vi "2d queue - Copia.vi"() -> ()   [LabVIEW 2020]
uses:
  control/Data Form.ctl
  control/fgv.ctl
  control/file structure.ctl
  <vilib>/Analysis/1siggen.llb/Ramp Pattern by Samples.vi
  queue/Front Panel Message Queue.lvlib
  <vilib>/Analysis/NI_AALBase.lvlib
panel:
  out "XY Graph":cluster{"Ramp Pattern":dbl[], dbl[]}(graph)
  out "Data Loaded":dbl[][](array[numeric])
  out "Data Form":T1
  out "error out":errorcluster
  in  "error in":errorcluster
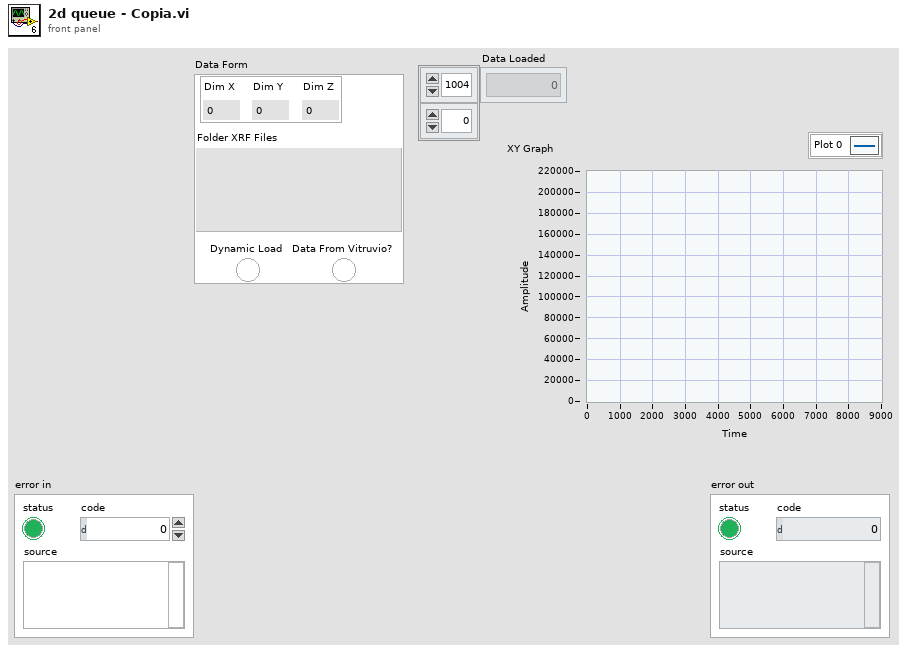
[diagram p1: front panel]
types:
  T1 = typedef "Data Form.ctl" = cluster{"Dimensions":cluster{"Dim X":i32, "Dim Y":i32, "Dim Z":i32}, "Folder XRF Files":path, "Dynamic Load":bool, "Data From Vitruvio?":bool}
  T2 = typedef "Front Panel Message Queue.lvlib/2d3d Message Queues.ctl" = cluster{"Main":refnum<queue>, "2d":refnum<queue>, "3d":refnum<queue>}
  T3 = typedef "fgv.ctl" = enum16{"initialize", "get data", "set data"}
  T4 = typedef "file structure.ctl" = cluster{"Colonna":i32, "Offset Righe":i32, "Coda Righe":i32, "Transpose":bool}
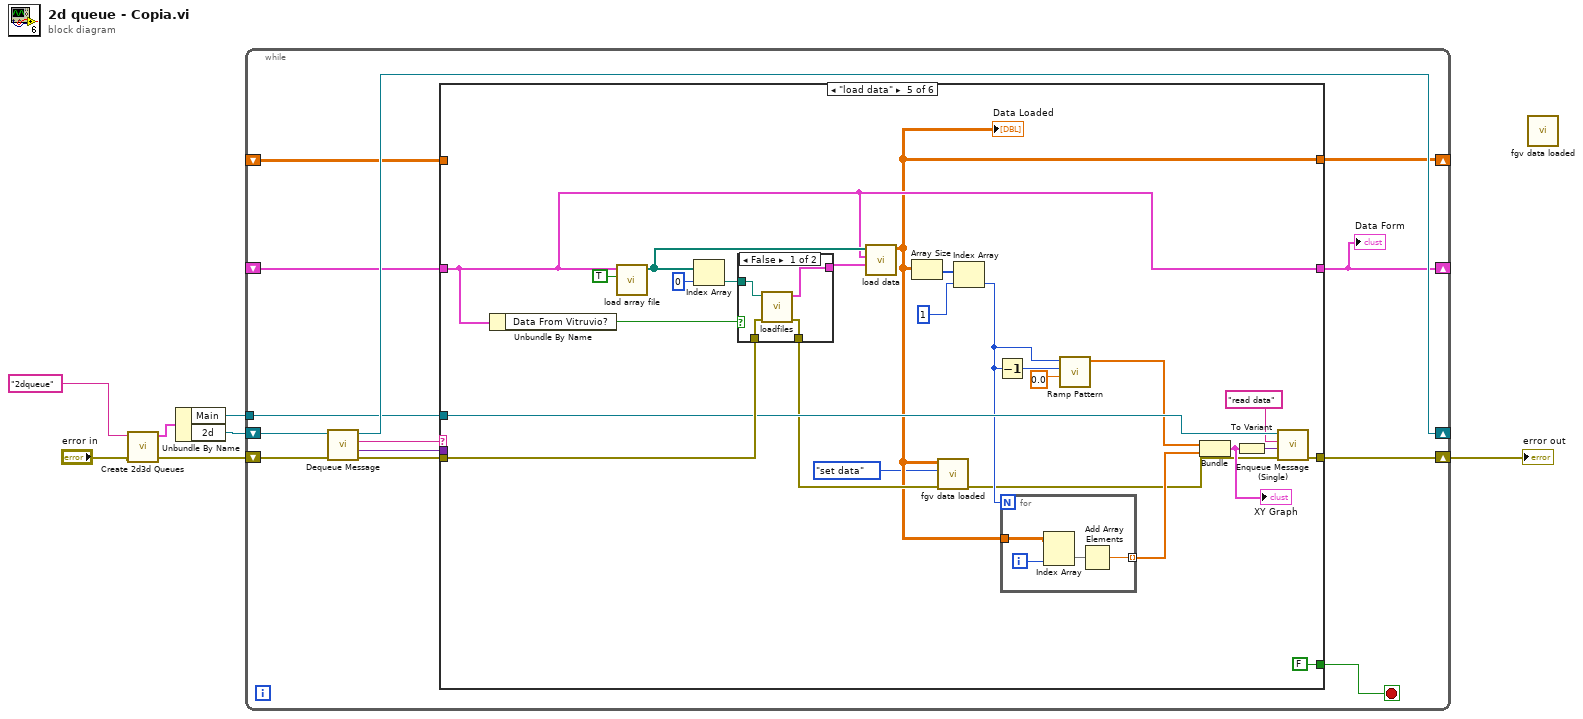
[diagram p0: block diagram]
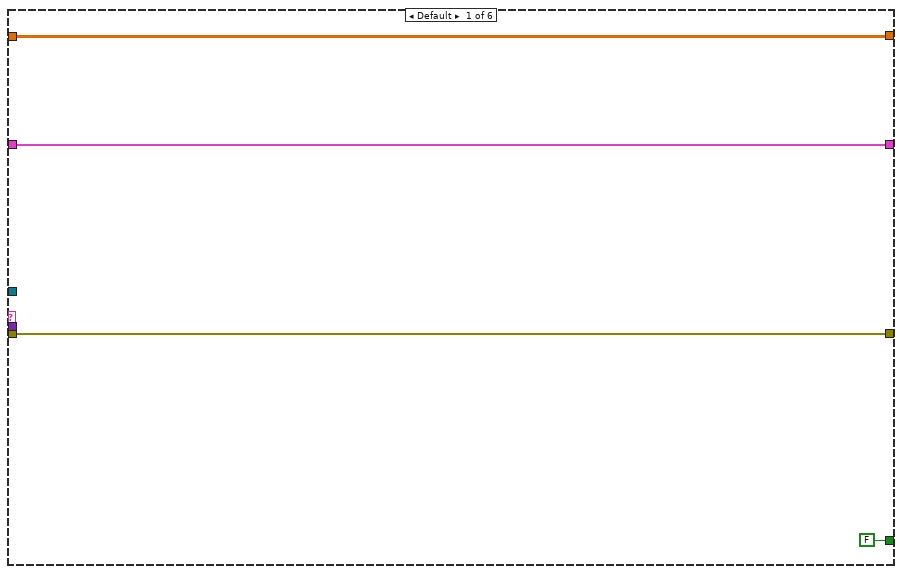
[diagram p2: hidden frame]
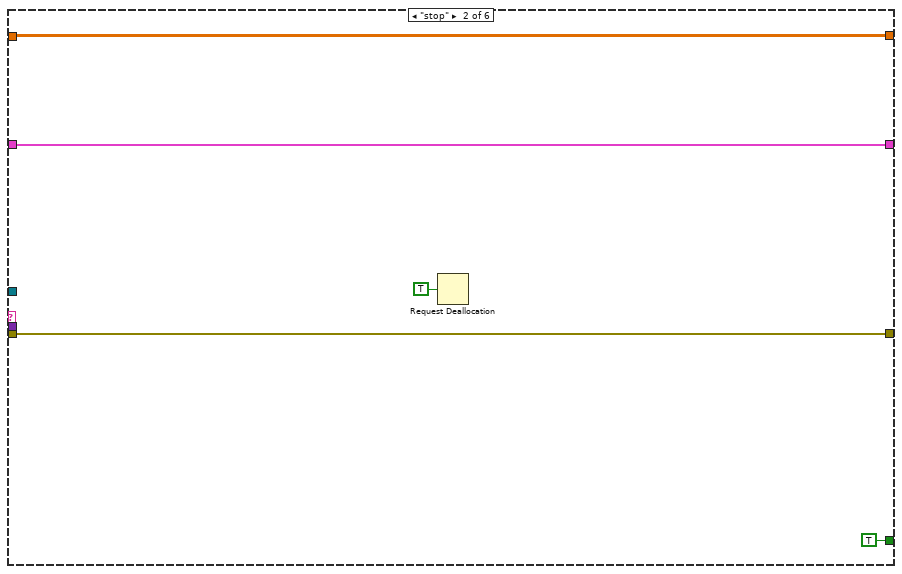
[diagram p3: hidden frame]
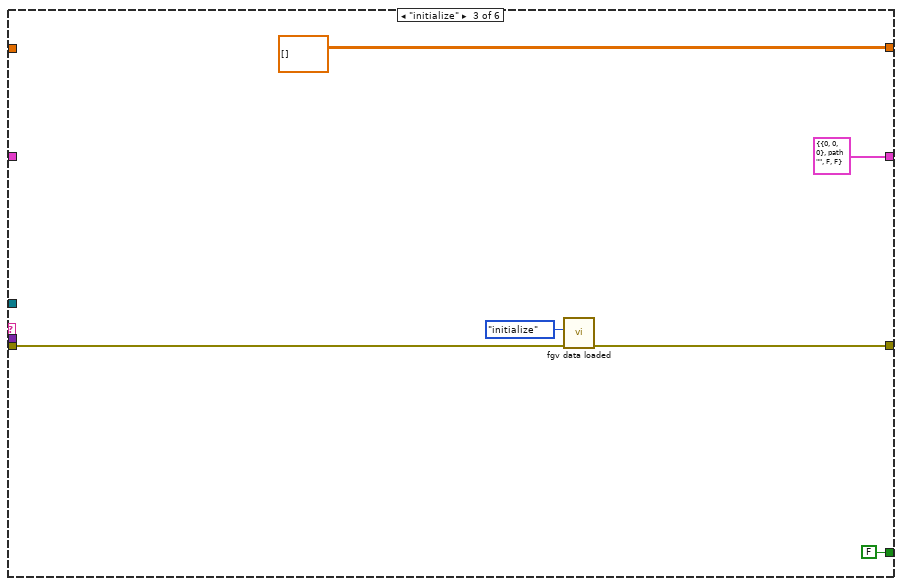
[diagram p4: hidden frame]
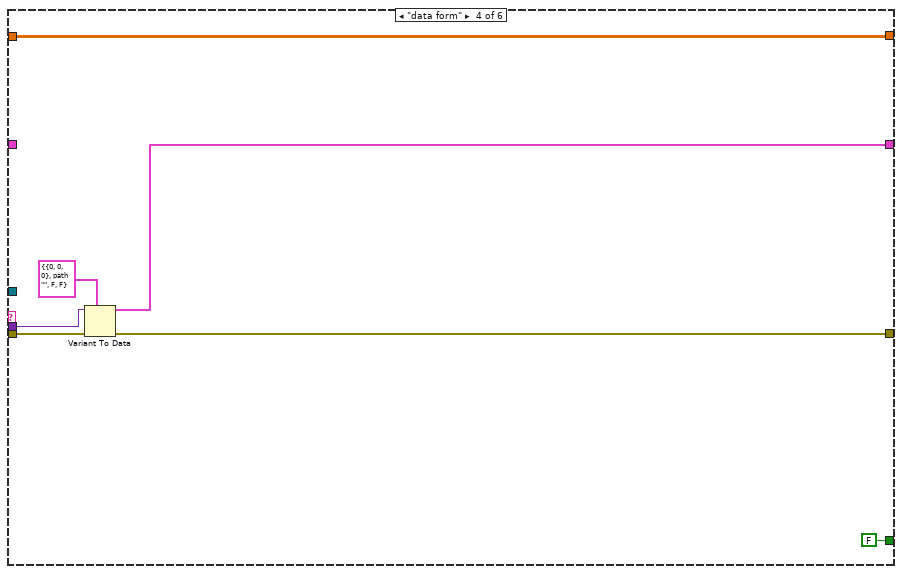
[diagram p5: hidden frame]
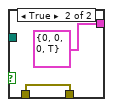
[diagram p6: hidden frame]
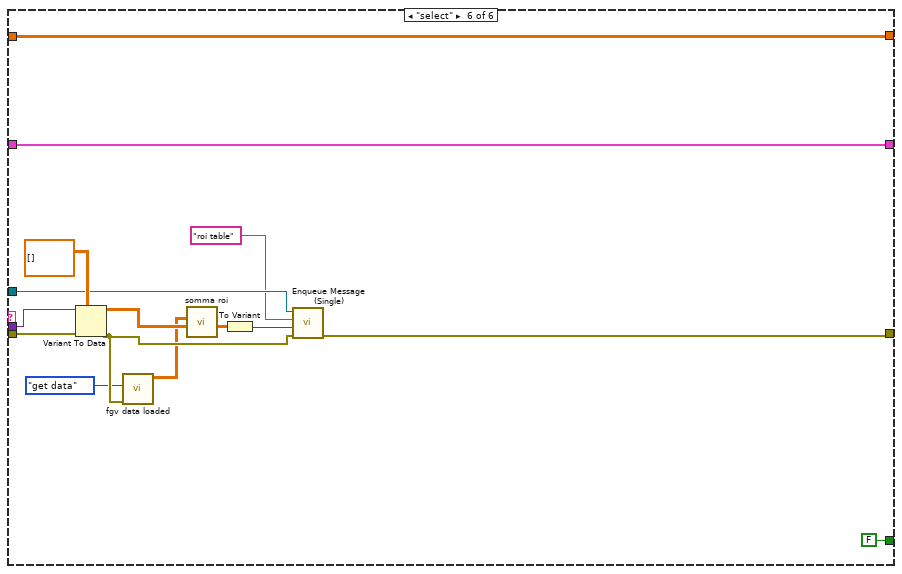
[diagram p7: hidden frame]
diagram:
  n1 = call "Create 2d3d Queues.vi"("error in (no error)"="error in", "name"="2dqueue") -> ("error out"=w4:errorcluster, "Message Queues"=w2:T2)  [unwired: 8 in]
  n2 = Unbundle By Name(w2) -> ("Main"=w1:refnum<queue>, "2d"=w7:refnum<queue>)
  n3 = while {
    shift-right: [w17] -> _
    shift-left: w7 -> [w19]
    shift-right: [w14] -> w6
    shift-left: w4 -> [w20]
    shift-right: [w11] -> _
    shift-left: _ -> [w12]
    shift-right: [w10] -> _
    shift-left: _ -> [w9]
    tunnel: w1 -> [w8]
    stop <- w15 stop-if-true
    n4 = call "Dequeue Message.vi"("error in (no error)"=w20, "Message Queue"=w19) -> ("error out"=w18:errorcluster, "Message Data"=w13:variant, "Message"=w16:string, "dup Message Queue"=w17:refnum<queue>)  [unwired: 5 in, 1 out]
    n5 = case shown="\"load data\"" w16 {
      tunnel: w18 -> [w23 w28 w31 w42 w63 w91]
      tunnel: [FALSE TRUE FALSE FALSE FALSE FALSE] -> w15
      tunnel: [w23 w28 w30 w38 w58 w83] -> w14
      tunnel: w13 -> [_ _ _ w41 _ w90]
      tunnel: [w22 w27 T1 {"Dimensions"={"Dim X"=0, "Dim Y"=0, "Dim Z"=0}, "Folder XRF Files"=path "", "Dynamic Load"=FALSE, "Data From Vitruvio?"=FALSE} ("Data Form") w39 w54 w82] -> w11
      tunnel: w12 -> [w22 w27 _ _ w54 w82]
      tunnel: [w21 w26 dbl[][] [] ("Data Loaded") w36 w44 w78] -> w10
      tunnel: w9 -> [w21 w26 _ w36 _ w78]
      tunnel: w8 -> [_ _ _ _ w57 w85]
      frame Default {
      }
      frame "stop" {
        n6 = Request Deallocation(TRUE ("flag")) -> ()
      }
      frame "initialize" {
        n7 = call "fgv data loaded.vi"("error in"=w31, "type"=fgv."initialize") -> ("error out"=w30:errorcluster)  [unwired: 8 in, 1 out]
      }
      frame "data form" {
        n8 = Variant To Data(error in=w42, type=T1 {"Dimensions"={"Dim X"=0, "Dim Y"=0, "Dim Z"=0}, "Folder XRF Files"=path "", "Dynamic Load"=FALSE, "Data From Vitruvio?"=FALSE} ("Data Form"), Variant=w41) -> (data=w39:T1, error out=w38:errorcluster)
      }
      frame "load data" {
        n9 = Unbundle By Name(w54) -> ("Data From Vitruvio?"=w53:bool)
        n10 = call "load array file.vi"("2d?"=TRUE, "Data Form"=w54) -> ("File Array Out"=w62:path[])  [unwired: 9 in]
        n11 = Index Array(array=w62, index=0) -> (element=w64:path)
        n12 = case shown="False" w53 {
          tunnel: w64 -> [w69 _]
          tunnel: w63 -> [w71 w73]
          tunnel: [w68 T4 {"Colonna"=0, "Offset Righe"=0, "Coda Righe"=0, "Transpose"=TRUE} ("File Structure")] -> w61
          tunnel: [w70 w73] -> w46
          frame False {
            n13 = call "loadfiles.vi"("Error In"=w71, "First Spectrum"=w69) -> ("Error Out"=w70:errorcluster, "File Structure"=w68:T4)  [unwired: 8 in]
          }
          frame True {
          }
        }
        n14 = call "load data.vi"("File Structure"=w61, "Data Form"=w54, "File Array In"=w62) -> ("Data Loaded"=w44:dbl[][])  [unwired: 8 in]
        "Data Loaded" <- w44
        n15 = Array Size(array=w44) -> (size(s)=w60:i32[])
        n16 = call "fgv data loaded.vi"("error in"=w46, "type"=fgv."set data", "New Data"=w44) -> ("error out"=w45:errorcluster)  [unwired: 7 in, 1 out]
        n17 = Index Array(array=w60, index=1) -> (element=w50:i32)
        n18 = Decrement(x=w50) -> (x-1=w52:i32)
        n19 = for {
          N: w50 -> [_]
          tunnel: w44 -> [w76]
          tunnel: [w74] -> w48 mode=indexing
          i -> [w75]
          n20 = Index Array(array=w76, index (col)=w75) -> (element=w77:dbl[])  [unwired: 1 in]
          n21 = Add Array Elements(numeric array=w77) -> (sum=w74:dbl)
        }
        n22 = call-poly <vilib>:"Ramp Pattern.vi"("start"=0.0, "end"=w52, "samples"=w50) -> ("Ramp Pattern"=w49:dbl[])  [unwired: 7 in, 1 out]
        n23 = Bundle("Ramp Pattern"=w49, w48) -> (w47:cluster{"Ramp Pattern":dbl[], dbl[]})  [unwired: 1 in]
        "XY Graph" <- w47
        n24 = To Variant(anything=w47) -> (Variant=w55:variant)
        n25 = call "Enqueue Message (Single).vi"("error in (no error)"=w45, "Message Data"=w55, "Message"="read data", "Message Queue"=w57) -> ("error out"=w58:errorcluster)  [unwired: 6 in, 1 out]
      }
      frame "select" {
        n26 = Variant To Data(error in=w91, type=dbl[][] [] ("ROIs Min Max"), Variant=w90) -> (data=w88:dbl[][], error out=w81:errorcluster)
        n27 = call "fgv data loaded.vi"("error in"=w81, "type"=fgv."get data") -> ("Data Loaded"=w79:dbl[][])  [unwired: 8 in, 1 out]
        n28 = call "somma roi.vi"("ROIs Min Max"=w88, "Data Loaded"=w79) -> ("ROIs Array Out"=w87:dbl[][])  [unwired: 9 in]
        n29 = To Variant(anything=w87) -> (Variant=w86:variant)
        n30 = call "Enqueue Message (Single).vi"("error in (no error)"=w81, "Message Data"=w86, "Message"="roi table", "Message Queue"=w85) -> ("error out"=w83:errorcluster)  [unwired: 6 in, 1 out]
      }
    }
    "Data Form" <- w11
  }
  "error out" <- w6
  n31 = call "fgv data loaded.vi"() -> ()  [unwired: 10 in, 2 out]
